vi "Scan Modules.vi"(8 "error in (no error)":errorcluster, 11 "Project In":refnum<class "Project.lvclass">) -> (0 "error out":errorcluster, 3 "Project Out":refnum<class "Project.lvclass">)   [LabVIEW 2019, in "Panther Dashboard.lvlib" / "Project.lvclass"]
uses:
  Project.lvclass
  Project.lvclass/Project.ctl
  Library/Library.lvclass/Library.ctl
  Library/Read Library Name.vi
  Read Main App Inst Ref.vi
  Read Libraries.vi
  Write Libraries.vi
  Library/Library.lvclass
  Panther Dashboard/Panther Dashboard.lvlib
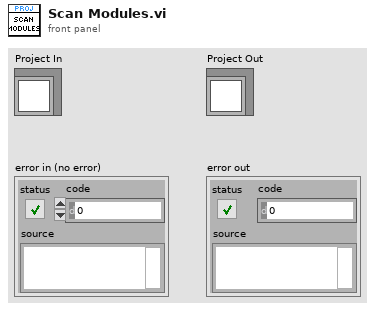
[diagram p1: front panel]
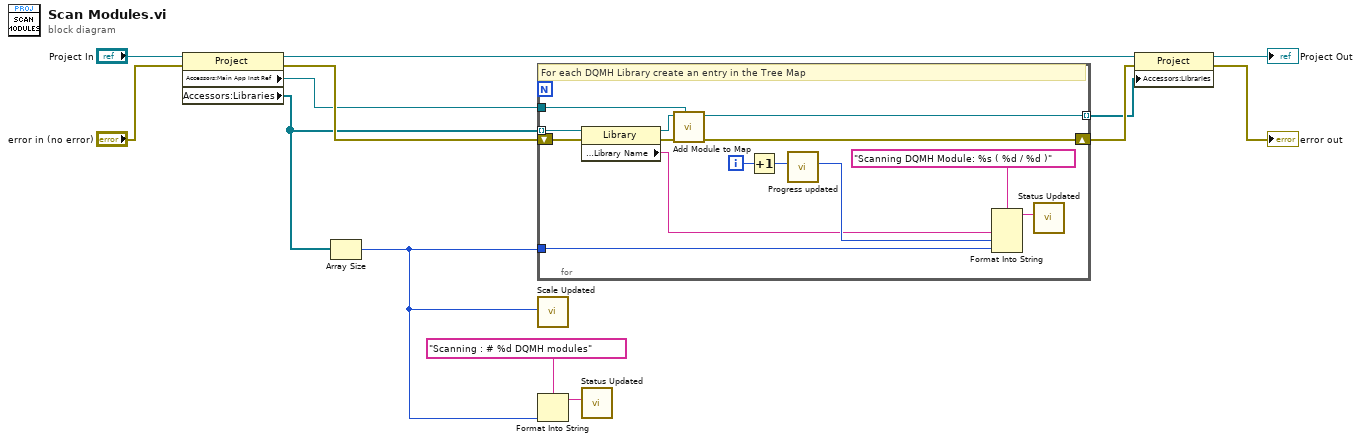
[diagram p0: block diagram]
diagram:
  n1 = property class="Project"(reference="Project In", error in="error in (no error)") -> (reference out=w5:refnum<class "Project.lvclass">, error out=w12:errorcluster, "Accessors:Main App Inst Ref"=w1:refnum<vi>, "Accessors:Libraries"=w2:refnum<class "Library.lvclass">[])
  n2 = Array Size(array=w2) -> (size(s)=w7:i32)
  n3 = for {
    tunnel: w7 -> [w22]
    tunnel: w1 -> [w18]
    tunnel: w2 -> [w17] mode=indexing
    tunnel: [w16] -> w3 mode=indexing
    shift-right: [w24] -> w11
    shift-left: w12 -> [w26]
    i -> [w23]
    # "For each DQMH Library create an entry in the Tree Map"
    n4 = property class="Library"(reference=w17, error in=w26) -> (reference out=w15:refnum<class "Library.lvclass">, error out=w25:errorcluster, "Accessors:Library Name"=w14:string)
    n5 = call "Add Module to Map.vi"("App Ref"=w18, "error in"=w25, "Library In"=w15) -> ("error out"=w24:errorcluster, "Library Out"=w16:refnum<class "Library.lvclass">)  [unwired: 7 in]
    n6 = Increment(x=w23) -> (x+1=w19:i32)
    n7 = call "Progress updated.vi"("Progress"=w19) -> ()  [unwired: 10 in, 1 out]
    n8 = Format Into String(format string="Scanning DQMH Module: %s ( %d / %d )", w14, w19, w22) -> (resulting string=w20:string)  [unwired: 2 in, 1 out]
    n9 = call "Status Updated.vi"("Status"=w20) -> ()  [unwired: 10 in, 1 out]
  }
  n10 = call "Scale Updated.vi"("Scale Max"=w7) -> ()  [unwired: 10 in, 1 out]
  n11 = Format Into String(format string="Scanning : # %d DQMH modules", w7) -> (resulting string=w9:string)  [unwired: 2 in, 1 out]
  n12 = call "Status Updated.vi"("Status"=w9) -> ()  [unwired: 10 in, 1 out]
  n13 = property class="Project"(reference=w5, error in=w11, "Accessors:Libraries"=w3) -> (reference out=→"Project Out":refnum<class "Project.lvclass">, error out=→"error out":errorcluster)
